vi "Update FIFO Header.vi"(11 "CIFChannels in":refnum<class "CIFChannels.lvclass">) -> (3 "CIFChannels out":refnum<class "CIFChannels.lvclass">)   [LabVIEW 2021, in "CIFChannels.lvclass"]
uses:
  CIFChannels.lvclass
  CIFChannels.lvclass/CIFChannels.ctl
  <vilib>/CIF Foundation/CIF Utilities/Time/System Time/LabVIEW Time to TAI Time.vi
  <vilib>/CIF Foundation/CIF Utilities/Time/Time_CIF_U.lvlib
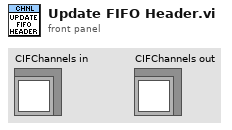
[diagram p1: front panel]
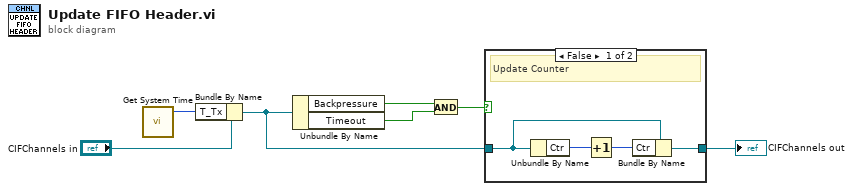
[diagram p0: block diagram]
diagram:
  n1 = call <vilib>:"Get System Time.vi"() -> ("Time (ns)"=w3:i64)  [unwired: 5 in]
  n2 = Bundle By Name(cluster="CIFChannels in", "T_Tx"=w3) -> (w4:refnum<class "CIFChannels.lvclass">)
  n3 = Unbundle By Name(w4) -> ("Backpressure"=w7:bool, "Timeout"=w6:bool)
  n4 = And(x=w7, y=w6) -> (x .and. y?=w5:bool)
  n5 = case shown="False" w5 {
    tunnel: w4 -> [w11 w12]
    tunnel: [w10 w12] -> w1
    frame False {
      # "Update Counter"
      n6 = Unbundle By Name(w11) -> ("Ctr"=w9:u64)
      n7 = Increment(x=w9) -> (x+1=w8:u64)
      n8 = Bundle By Name(cluster=w11, "Ctr"=w8) -> (w10:refnum<class "CIFChannels.lvclass">)
    }
    frame True {
      # "Retry last packet"
    }
  }
  "CIFChannels out" <- w1
